vi "rotate2body.vi"(3 "psi":dbl, 4 "2":dbl, 5 "1":dbl) -> (0 "2_body":dbl, 2 "1_body":dbl)   [LabVIEW 2014]
uses:
  <vilib>/imath/engines/lvmath2/RunTimeEngine/ArithmeticOperatorToken/NIMS_ArithmeticOperator_multmx(M,CV).vi
  <instcachedir>/0/NIMS_ArithmeticOperator_multmx(M,CV)_787B4652E60B4C52835A7FB23671E425.lvgen/NIMS_ArithmeticOperator_multmx(M,CV)_787B4652E60B4C52835A7FB23671E425_000.vi
  <vilib>/imathl/engines/lvmath/Functions/Error Handling/Create Error.vi
  <vilib>/imath/engines/lvmath2/RunTimeEngine/IndexRead/NIMS M(S).vi
  <instcachedir>/0/NIMS M(S)_B826C018497E4940AE96BD27B540B6FB.lvgen/NIMS M(S)_B826C018497E4940AE96BD27B540B6FB_000.vi
  <vilib>/imath/engines/lvmath2/RunTimeEngine/NodeEndStatement/NIMS_NodeEndStatement_Output.vi
  <instcachedir>/0/NIMS_NodeEndStatement_Output_53EC0D466D134D7ABD903AC30B43404B.lvgen/NIMS_NodeEndStatement_Output_53EC0D466D134D7ABD903AC30B43404B_001.vi
  <vilib>/imath/engines/lvmath2/RunTimeEngine/ErrorHandling/NIMS_Finalize Error.vi
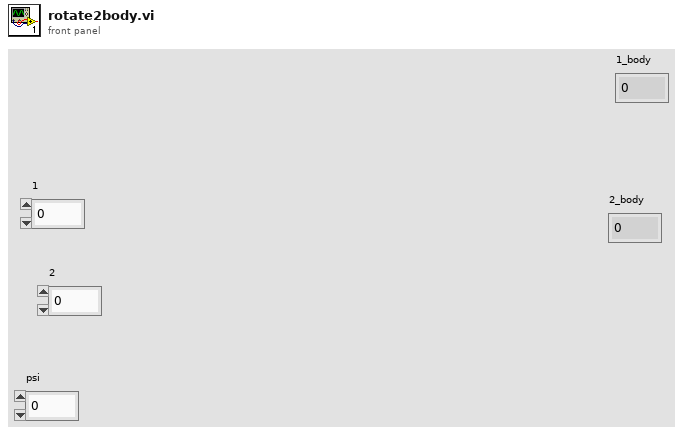
[diagram p1: front panel]
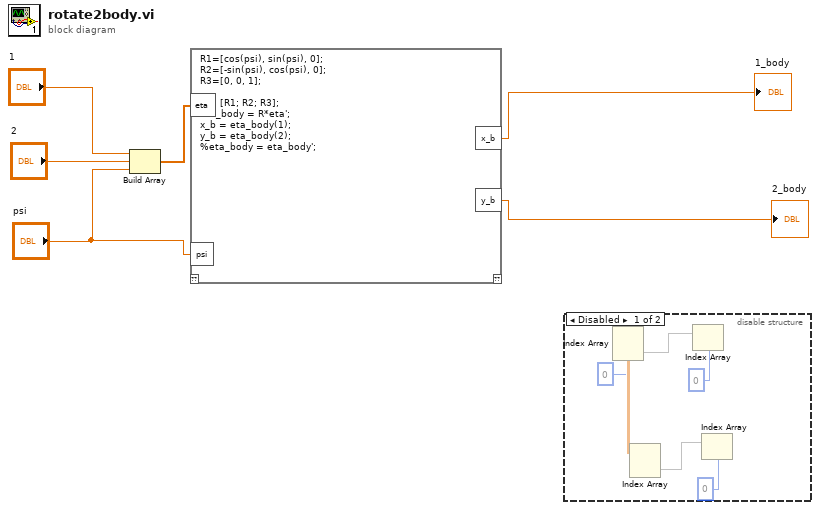
[diagram p0: block diagram]
diagram:
  n1 = Build Array("1", "2", "psi") -> (w4:dbl[])
  n2 = mathscript code="R1=[cos(psi), sin(psi), 0];\nR2=[-sin(psi), cos(psi), 0];\nR3=[0, 0, 1];\n\nR = [R1; R2; R3];\neta_body = R*eta';\nx_b = eta_body(1);\ny_b = eta_body(2);\n%eta_body = eta_body';"("eta"=w4, "psi"="psi") -> ("x_b"=→"1_body":dbl, "y_b"=→"2_body":dbl)  [unwired: 1 in, 1 out]
  n3 = disable-structure shown="Disabled" {
    frame Disabled {
      n4 = Index Array(index (row)=0 ("index")) -> (array=w12:dbl[][], element=w11)  [unwired: 1 in]
      n5 = Index Array(array=w12) -> (element=w10)  [unwired: 2 in]
      n6 = Index Array(array=w11, index=0) -> ()  [unwired: 1 out]
      n7 = Index Array(array=w10, index=0) -> ()  [unwired: 1 out]
    }
    frame Enabled {
    }
  }
